vi "LX.vi"() -> ()   [LabVIEW 2020]
panel:
  in  "LX":dbl
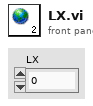
[diagram p1: front panel]
diagram:
